vi "Wait.vi"(11 "milliseconds to wait":u32) -> (3 "Boolean":bool=TRUE)   [LabVIEW 2018]
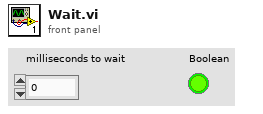
[diagram p1: front panel]
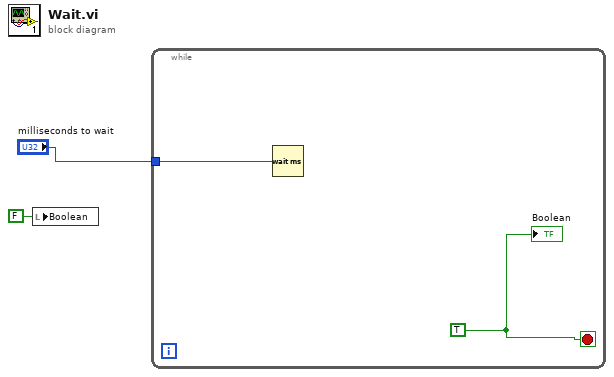
[diagram p0: block diagram]
diagram:
  n1 = local write "Boolean"(FALSE ("Boolean")) -> ()
  n2 = while {
    tunnel: "milliseconds to wait" -> [w4]
    stop <- w3 stop-if-true
    w3 = TRUE
    n3 = Wait (ms)(milliseconds to wait=w4) -> ()  [unwired: 1 out]
    "Boolean" <- w3
  }
